vi "To Center and Span (bare).vi"(4 "stop":dbl, 6 "start":dbl) -> (0 "span":dbl, 2 "center":dbl)   [LabVIEW 2023]
doc: "Takes two bare numbers that indicate the beginning and end of a range and returns the average (\"center\") and difference (\"span\") of the two numbers."
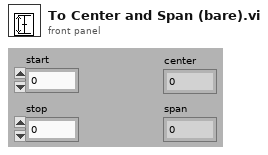
[diagram p1: front panel]
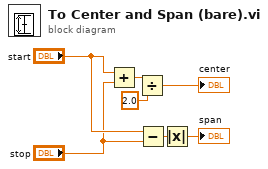
[diagram p0: block diagram]
diagram:
  n1 = Add(x="start", y="stop") -> (x+y=w7:dbl)
  n2 = Divide(x=w7, y=2.0) -> (x/y=→"center":dbl)
  n3 = Subtract(x="start", y="stop") -> (x-y=w2:dbl)
  n4 = Absolute Value(x=w2) -> (abs(x)=→"span":dbl)
